vi "Raw to I16.vi"(8 "error in (no error)":errorcluster, 10 "Raw data":string, 11 "RP I-V Driver in":refnum<class "RP I-V Driver.lvclass">) -> (0 "error out":errorcluster, 1 "Current read position":i32, 2 "Data out":i16[][](array[numeric]), 3 "RP I-V Driver out":refnum<class "RP I-V Driver.lvclass">, 4 "Finished":bool)   [LabVIEW 2016, in "RP I-V Driver.lvclass"]
uses:
  RP I-V Driver.lvclass
  C:/github/NHMFL_Core/Libraries/Instruments/Pulse Driver/Pulse Driver.lvclass
  Instruments/Pulse Driver/Pulse Driver.lvclass/Pulse Driver.ctl
  Instruments/Pulse Driver/Write Scaling coefficients.vi
  Instruments/Pulse Driver/Read Current read position.vi
  Instruments/Pulse Driver/Read Scaling coefficients.vi
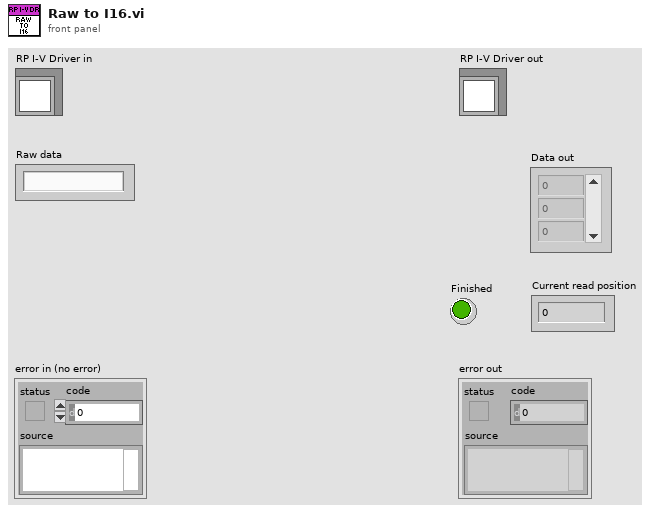
[diagram p1: front panel]
types:
  T1 = enum16{"big-endian, network order", "native, host order", "little-endian"}
  T2 = typedef "RP I-V Configuration.ctl" = cluster{"I-V parameters":T3, "Ranges":dbl[], "Pre-trigger duration":dbl, "Post-trigger duration":dbl, "Output delay":dbl}
  T3 = typedef "I-V parameters.ctl" = cluster{"Start magnitude":dbl, "Magnitude increment":dbl, "Number of pulses":i32, "Baseline length":i32, "Ramp length":i32, "Top  length":i32, "Threshold ":dbl, "Processing delay":u16, "Valhalla range":dbl, "Interpolation":i32}
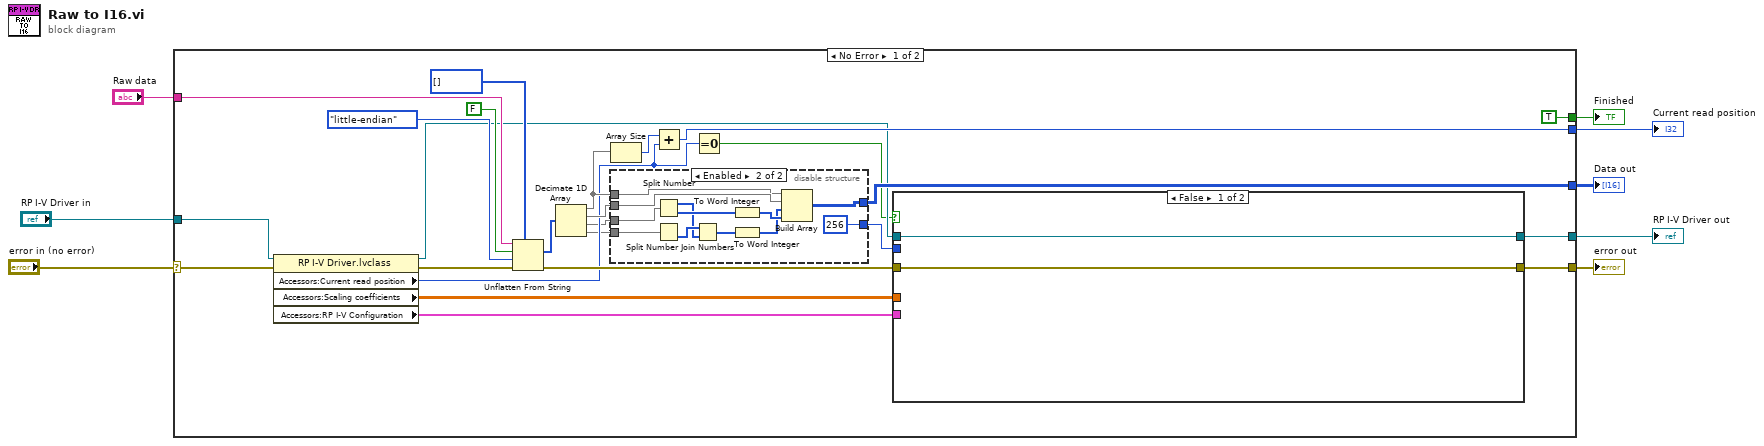
[diagram p0: block diagram]
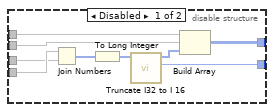
[diagram p2: hidden frame]
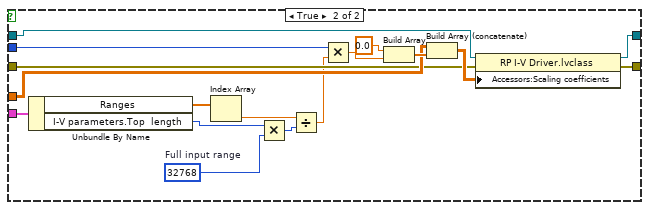
[diagram p3: hidden frame]
diagram:
  n1 = case shown="No Error" "error in (no error)" {
    selector: "error in (no error)" -> [w26 w75]
    tunnel: [w16 w75] -> w5
    tunnel: [w18 w74] -> w7
    tunnel: "RP I-V Driver in" -> [w22 w74]
    tunnel: "Raw data" -> [w28 _]
    tunnel: [w25 _] -> w4
    tunnel: [w24 _] -> w3
    tunnel: [TRUE ("Finished") _] -> w2
    frame No Error {
      n2 = property class="RP I-V Driver.lvclass"(reference=w22, error in=w26) -> (reference out=w19:refnum<class "RP I-V Driver.lvclass">, error out=w27:errorcluster, "Accessors:Current read position"=w11:i32, "Accessors:Scaling coefficients"=w20:dbl[][], "Accessors:RP I-V Configuration"=w21:T2)
      n3 = Unflatten From String(type=i16[] [], binary string=w28, data includes array or string size? (T)=FALSE, byte order (0:big-endian, network order)=T1."little-endian", error in (no error)=w27) -> (value=w29:i16[], error out=w17:errorcluster)  [unwired: 1 out]
      n4 = Decimate 1D Array(w29) -> (w14:i16[], w33:i16[], w9:i16[], w10:i16[])
      n5 = Array Size(array=w14) -> (size(s)=w13:i32)
      n6 = disable-structure shown="Enabled" {
        disable-tunnel: w33 -> [w42 w54]
        disable-tunnel: [w41 w53] -> w24
        disable-tunnel: [w39 256 ("divider")] -> w15
        disable-tunnel: w14 -> [w38 w52]
        disable-tunnel: w10 -> [w36 w47]
        disable-tunnel: w9 -> [w35 w50]
        frame Disabled {
          n7 = Join Numbers(hi=w36, lo=w35) -> ((hi.lo)=w34:u32[])
          n8 = To Long Integer(number=w34) -> (32bit integer=w37:i32[])
          n9 = call "Truncate I32 to I 16.vi"("Data"=w37) -> ("divider"=w39:i32, "Data out"=w40:i16[])  [unwired: 8 in, 1 out]
          n10 = Build Array(w38, w42, w40) -> (w41:i16[][])
        }
        frame Enabled {
          n11 = Split Number(x=w50) -> (hi(x)=w45:u8[], lo(x)=w49:u8[])
          n12 = Split Number(x=w47) -> (lo(x)=w46:u8[])  [unwired: 1 out]
          n13 = Join Numbers(hi=w46, lo=w45) -> ((hi.lo)=w44:u16[])
          n14 = To Word Integer(number=w49) -> (16bit integer=w48:i16[])
          n15 = To Word Integer(number=w44) -> (16bit integer=w43:i16[])
          n16 = Build Array(w52, w54, w43, w48) -> (w53:i16[][])
        }
      }
      n17 = Add(x=w13, y=w11) -> (x+y=w25:i32)
      n18 = Equal To 0?(x=w11) -> (x = 0?=w12:bool)
      n19 = case shown="False" w12 {
        tunnel: w21 -> [_ w65]
        tunnel: w20 -> [_ w64]
        tunnel: w19 -> [w55 w63]
        tunnel: [w55 w62] -> w18
        tunnel: w17 -> [w56 w61]
        tunnel: [w56 w60] -> w16
        tunnel: w15 -> [_ w57]
        frame False {
        }
        frame True {
          w70 = 32768  # Full input range
          n20 = Unbundle By Name(w65) -> ("Ranges"=w68:dbl[], "I-V parameters.Top  length"=w66:i32)
          n21 = Index Array(array=w68) -> (element=w69:dbl)  [unwired: 1 in]
          n22 = Multiply(x=w66, y=w70) -> (x*y=w71:i32)
          n23 = Divide(x=w69, y=w71) -> (x/y=w58:dbl)
          n24 = Multiply(x=w57, y=w58) -> (x*y=w59:dbl)
          n25 = Build Array(0.0 ("element"), w59) -> (w72:dbl[])
          n26 = Build Array (concatenate)(w64, w72) -> (w67:dbl[][])
          n27 = property class="RP I-V Driver.lvclass"(reference=w63, error in=w61, "Accessors:Scaling coefficients"=w67) -> (reference out=w62:refnum<class "RP I-V Driver.lvclass">, error out=w60:errorcluster)
        }
      }
    }
    frame Error {
    }
  }
  "error out" <- w5
  "RP I-V Driver out" <- w7
  "Finished" <- w2
  "Current read position" <- w4
  "Data out" <- w3
